vi "Post-Processing Main.vi"() -> ()   [LabVIEW 2019]
uses:
  Counts.ctl
  Post-Processing/State Data.ctl
  Post-Processing/File Entry.ctl
  Post-Processing/ADC Bounds.ctl
  <vilib>/Utility/sysdir.llb/System Directory Type.ctl
  Post-Processing/Muon Data Post-Processing.lvlib
panel:
  out "Total Duration":string
  in  "Display Type":enum16{"Both", "Nearest", "Largest"}(ring)
  out "Version Number":string
  out "Total Duration (s)":dbl
  in  "Count only matching 3-Events":bool=TRUE
  in  "File":string(combo)
  in  "Directory":path
  in  "Slave Slider":cluster{"Numeric":u16, "Numeric":u16}(slide)={"Numeric"=0, "Numeric"=1} scale=0.0..1023.0
  in  "Master Slider":cluster{"Numeric":u16, "Numeric":u16}(slide)={"Numeric"=0, "Numeric"=9} scale=0.0..1023.0
  out "Slave 'Histogram'":cluster{cluster{dbl, dbl}[]}[](graph)
  out "Master 'Histogram'":cluster{cluster{dbl, dbl}[]}[](graph)
  out "Event Counts":T1 {"Coincident Event Rate" format="%.4g"; "Single Slave Event Rate" format="%.4g"; "Single Master Event Rate" format="%.4g"}
  out "Event ADC Counts Graph":T2(graph)
  # "S-Min, Max"
  # "M-Min, Max"
  # "The histograms show both single and coincident values"
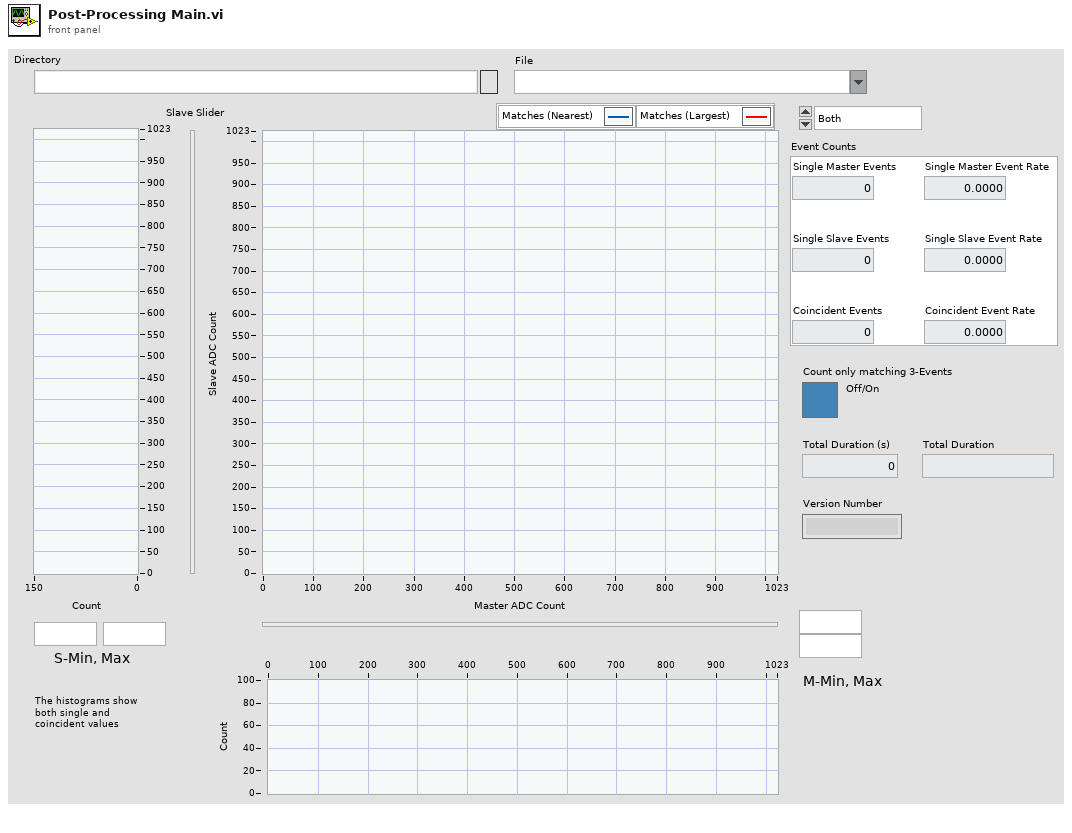
[diagram p1: front panel]
types:
  T1 = typedef "Counts.ctl" = cluster{"Single Master Events":i32, "Single Slave Events":i32, "Coincident Events":i32, "Single Master Event Rate":dbl, "Single Slave Event Rate":dbl, "Coincident Event Rate":dbl}
  T2 = cluster{"Matched ADC Values - Largest":cluster{"Master ADC Value":i32, "Slave ADC Value":i32}[]}[]
  T3 = enum32{"Invalid", "Standard", "Closed", "Hidden", "Minimized", "Maximized"}
  T4 = typedef "System Directory Type.ctl" = i32
  T5 = typedef "Muon Data Post-Processing.lvlib/State Data.ctl" = cluster{"Raw File Data":string, "Deduplicated String Array":string[][], "1-Entries":T6[], "2-Entries":T6[], "3-Entries":T6[], "Bounds":T7, "Matched ADC Values - Nearest":cluster{"Master ADC Value":i32, "Slave ADC Value":i32}[], "Match Entry Indices - Nearest":cluster{"Master Entry Index":i32, "Slave Entry Index":i32}[], "Filtered 1-Entries":T6[], "Filtered 2-Entries":T6[], "Filtered 3-Entries":T6[], "Total Duration":dbl, "Matched ADC Values - Largest":cluster{"Master ADC Value":i32, "Slave ADC Value":i32}[], "Match Entry Indices - Largest":cluster{"Master Entry Index":i32, "Slave Entry Index":i32}[]}
  T6 = typedef "Muon Data Post-Processing.lvlib/File Entry.ctl" = cluster{"Entry Index":i32, "PC Time":timestamp, "File Index":i32, "Arduino Time":i32, "ADC Value":i32, "Event Type":i32, "Detector":string}
  T7 = typedef "Muon Data Post-Processing.lvlib/ADC Bounds.ctl" = cluster{"M-Min":u16, "M-Max":u16, "S-Min":u16, "S-Max":u16}
  T8 = cluster{"Master ADC Value":i32, "Slave ADC Value":i32}[]
  T9 = cluster{"Matched ADC Values - Largest":cluster{"Master ADC Value":i32, "Slave ADC Value":i32}[]}
  T10 = cluster{"Matched ADC Values - Nearest":cluster{"Master ADC Value":i32, "Slave ADC Value":i32}[]}
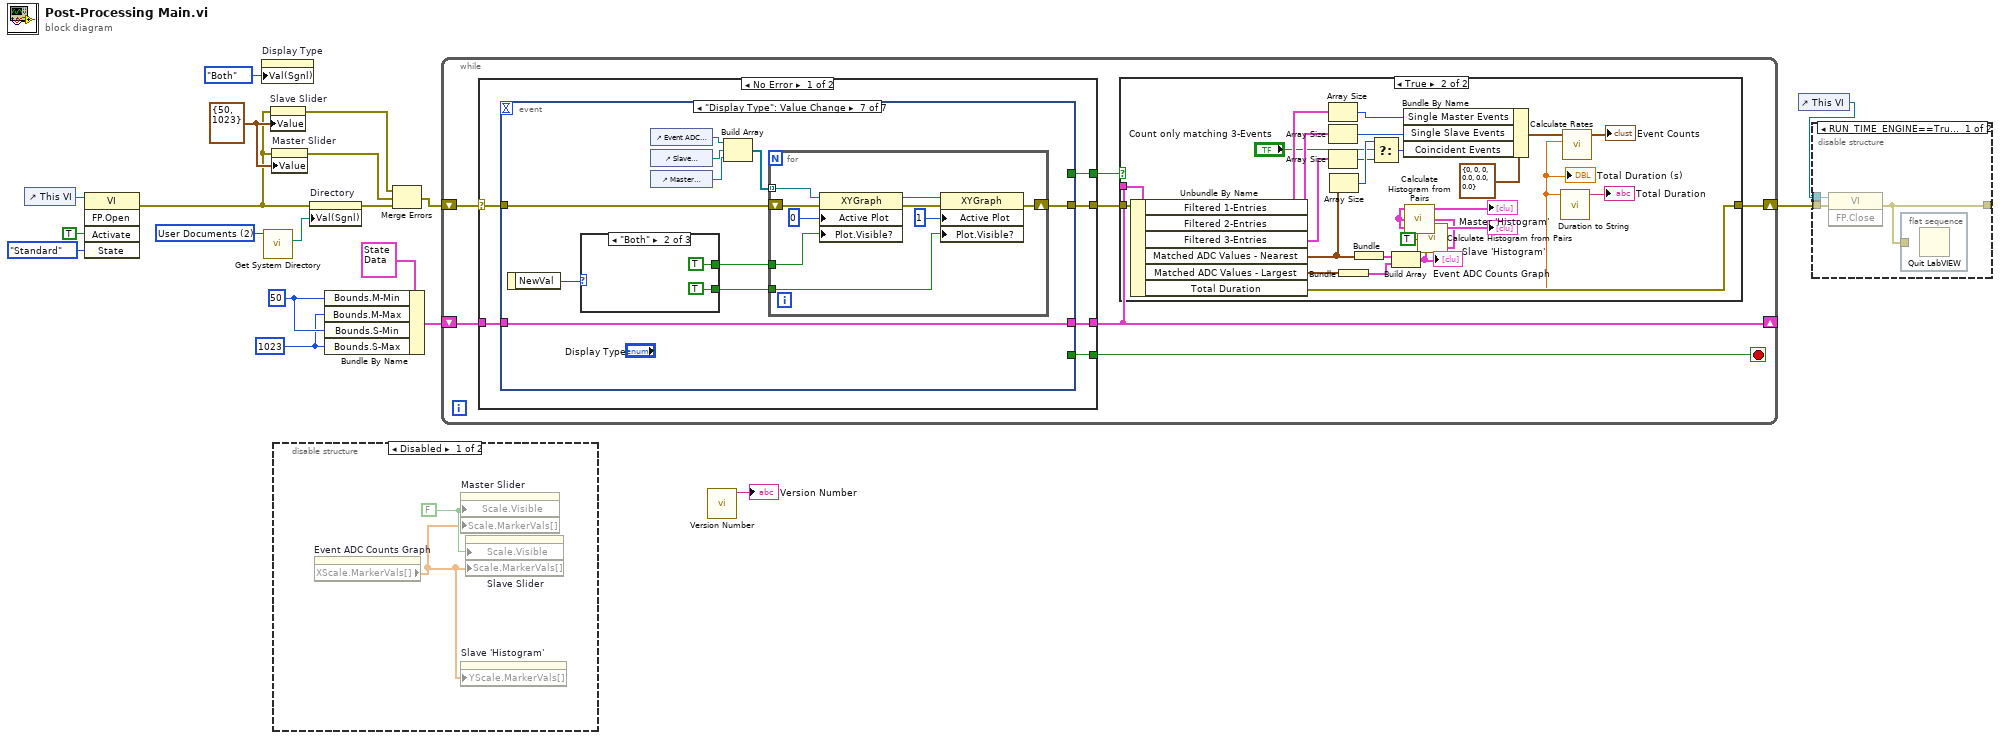
[diagram p0: block diagram]
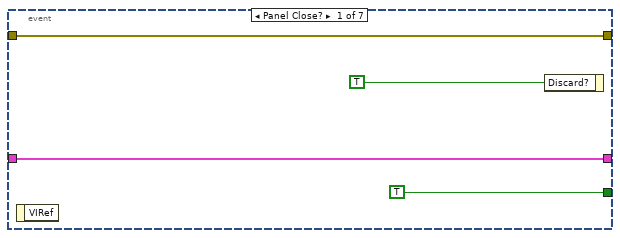
[diagram p3: hidden frame]
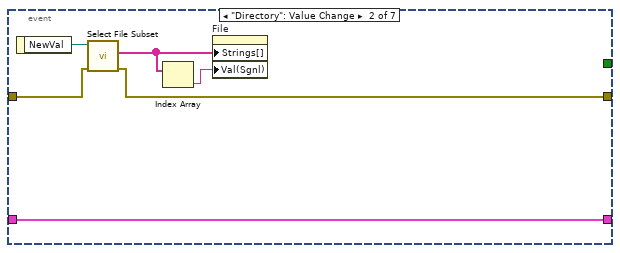
[diagram p4: hidden frame]
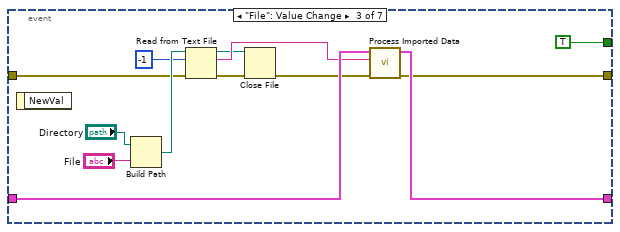
[diagram p5: hidden frame]
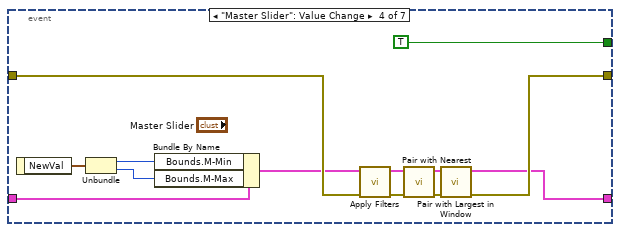
[diagram p6: hidden frame]
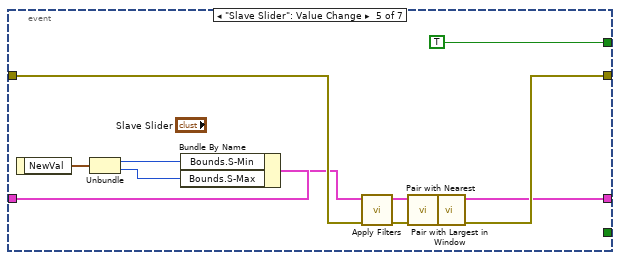
[diagram p7: hidden frame]
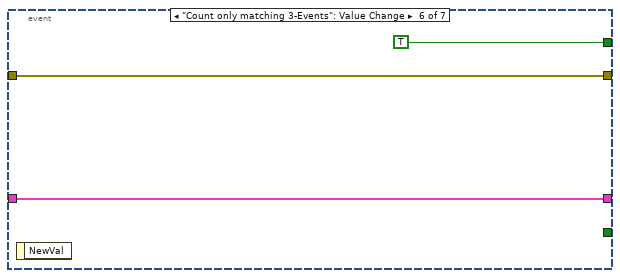
[diagram p8: hidden frame]
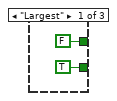
[diagram p9: hidden frame]
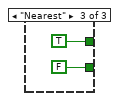
[diagram p10: hidden frame]
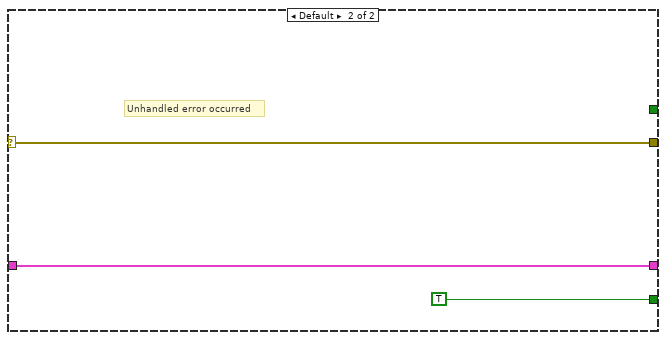
[diagram p11: hidden frame]
diagram:
  w11 = T4 2 items=["User Home"=0, "User Desktop"=1, "User Documents"=2, "User Application Data"=3, "User Preferences"=4, "User Temporary"=5, "Public Documents"=6, "Public Application Data"=7, "Public Preferences"=8, "Public Cache"=13, "System Core Libraries"=9, "System Installed Libraries"=10, "Application Files"=11, "Boot Volume Root"=12] ("system directory type")
  w12 = u16 1023 ("Bounds.M-Max")
  w13 = u16 50 ("Bounds.M-Min")
  w17 = cluster{"Numeric":u16, "Numeric":u16} {"Numeric"=50, "Numeric"=1023} ("Slave Slider")
  n1 = control-ref of="This VI"() -> (w9:refnum<vi>)
  n2 = invoke class="VI" method="FP.Open"(reference=w9, "Activate"=TRUE ("Activate?"), "State"=T3."Standard") -> (error out=w4:errorcluster)  [unwired: 2 in, 4 out]
  n3 = property on="Display Type" class="Enum (strict)"("Val(Sgnl)"=enum16{"Both", "Nearest", "Largest"}."Both" ("Value (Signaling)")) -> ()  [unwired: 2 in, 2 out]
  n4 = call <vilib>:"Get System Directory.vi"("system directory type"=w11) -> ("system directory"=w10:path)  [unwired: 10 in]
  n5 = property on="Slave Slider" class="Slide (strict)"(error in=w4, "Value"=w17) -> (error out=w16:errorcluster)  [unwired: 1 in, 1 out]
  n6 = property on="Master Slider" class="Slide (strict)"(error in=w4, "Value"=w17) -> (error out=w15:errorcluster)  [unwired: 1 in, 1 out]
  n7 = disable-structure shown="Disabled" {
    frame Disabled {
      w21 = FALSE ("Scale.Visible")
      n8 = property on="Event ADC Counts Graph" class="XYGraph (strict)"() -> ("XScale.MarkerVals[]"=w20:dbl[])  [unwired: 2 in, 2 out]
      n9 = property on="Master Slider" class="Slide (strict)"("Scale.Visible"=w21, "Scale.MarkerVals[]"=w20) -> ()  [unwired: 2 in, 2 out]
      n10 = property on="Slave 'Histogram'" class="XYGraph (strict)"("YScale.MarkerVals[]"=w20) -> ()  [unwired: 2 in, 2 out]
      n11 = property on="Slave Slider" class="Slide (strict)"("Scale.Visible"=w21, "Scale.MarkerVals[]"=w20) -> ()  [unwired: 2 in, 2 out]
    }
    frame Enabled {
    }
  }
  n12 = property on="Directory" class="Path"(error in=w4, "Val(Sgnl)"=w10) -> (error out=w19:errorcluster)  [unwired: 1 in, 1 out]
  n13 = Bundle By Name(cluster=T5 {"Raw File Data"="", "Deduplicated String Array"=[], "1-Entries"=[], "2-Entries"=[], "3-Entries"=[], "Bounds"={"M-Min"=0, "M-Max"=1023, "S-Min"=0, "S-Max"=1023}, "Matched ADC Values - Nearest"=[], "Match Entry Indices - Nearest"=[], "Filtered 1-Entries"=[], "Filtered 2-Entries"=[], "Filtered 3-Entries"=[], "Total Duration"=0.0, "Matched ADC Values - Largest"=[], "Match Entry Indices - Largest"=[]}, "Bounds.M-Min"=w13, "Bounds.M-Max"=w12, "Bounds.S-Min"=w13, "Bounds.S-Max"=w12) -> (w14:T5)
  n14 = Merge Errors(w16, w15, w19) -> (w3:errorcluster)
  n15 = while {
    shift-right: [w24] -> w6
    shift-left: w3 -> [w26]
    shift-right: [w28] -> _
    shift-left: w14 -> [w25]
    stop <- w27 stop-if-true
    n16 = case shown="No Error" w26 {
      selector: w26 -> [w33 w114]
      tunnel: [w34 TRUE] -> w27
      tunnel: [w32 w114] -> w23
      tunnel: w25 -> [w31 w112]
      tunnel: [w30 w112] -> w28
      tunnel: [w29 _] -> w22
      frame No Error {
        n17 = event shown="[6] \"Display Type\": Value Change" {
          selector: _ -> [_ _ _ _ _ _ _]
          dyn-events: _ -> [_ _ _ _ _ _ _]
          timeout: _ -> [_ _ _ _ _ _ _]
          tunnel: [TRUE _ _ _ _ _ _] -> w34
          tunnel: w33 -> [w36 w41 w52 w69 w83 w85 w94]
          tunnel: [w36 w40 w46 w60 w73 w85 w95] -> w32
          tunnel: w31 -> [w35 w39 w57 w68 w78 w84 w96]
          tunnel: [w35 w39 w48 w58 w71 w84 w96] -> w30
          tunnel: [_ _ TRUE TRUE TRUE TRUE _] -> w29
          event Panel Close? {
            n18 = event-data() -> ()  [unwired: 1 in, 1 out]
            n19 = event-data("Discard?"=TRUE) -> ()  [unwired: 1 in, 1 out]
          }
          event "Directory": Value Change {
            n20 = event-data() -> ("NewVal"=w43:path)  [unwired: 1 in]
            n21 = call "Select File Subset.vi"("error in"=w41, "Directory"=w43) -> ("error out"=w40:errorcluster, "File List"=w42:string[])  [unwired: 8 in]
            n22 = Index Array(array=w42) -> (element=w44:string)  [unwired: 1 in]
            n23 = property on="File" class="CmbBox"("Strings[]"=w42, "Val(Sgnl)"=w44) -> ()  [unwired: 2 in, 2 out]
          }
          event "File": Value Change {
            n24 = event-data() -> ()  [unwired: 1 in, 1 out]
            n25 = Build Path(base path="Directory", name or relative path="File") -> (appended path=w55:path)
            n26 = Read from Text File(file (use dialog)=w55, count=-1, error in=w52) -> (refnum out=w50:refnum<file>, text=w56:string, error out=w51:errorcluster)  [unwired: 1 in, 1 out]
            n27 = Close File(refnum=w50, error in=w51) -> (error out=w47:errorcluster)  [unwired: 1 out]
            n28 = call "Process Imported Data.vi"("error in (no error)"=w47, "Raw File Data"=w56, "State Data in"=w57) -> ("error out"=w46:errorcluster, "State Data out"=w48:T5)  [unwired: 7 in]
          }
          event "Master Slider": Value Change {
            n29 = event-data() -> ("NewVal"=w66:cluster{"Numeric":u16, "Numeric":u16})  [unwired: 1 in]
            n30 = Unbundle(w66) -> ("Numeric"=w65:u16, "Numeric"=w64:u16)
            n31 = Bundle By Name(cluster=w68, "Bounds.M-Min"=w65, "Bounds.M-Max"=w64) -> (w62:T5)
            n32 = call "Apply Filters.vi"("error in (no error)"=w69, "State in"=w62) -> ("error out"=w63:errorcluster, "State out"=w61:T5)  [unwired: 8 in]
            n33 = call "Pair with Nearest.vi"("error in (no error)"=w63, "State in"=w61) -> ("error out"=w70:errorcluster, "State out"=w59:T5)  [unwired: 8 in]
            n34 = call "Pair with Largest in Window.vi"("error in (no error)"=w70, "State in"=w59) -> ("error out"=w60:errorcluster, "State out"=w58:T5)  [unwired: 8 in]
          }
          event "Slave Slider": Value Change {
            n35 = event-data() -> ("NewVal"=w79:cluster{"Numeric":u16, "Numeric":u16})  [unwired: 1 in]
            n36 = Unbundle(w79) -> ("Numeric"=w81:u16, "Numeric"=w80:u16)
            n37 = Bundle By Name(cluster=w78, "Bounds.S-Min"=w81, "Bounds.S-Max"=w80) -> (w75:T5)
            n38 = call "Apply Filters.vi"("error in (no error)"=w83, "State in"=w75) -> ("error out"=w76:errorcluster, "State out"=w74:T5)  [unwired: 8 in]
            n39 = call "Pair with Nearest.vi"("error in (no error)"=w76, "State in"=w74) -> ("error out"=w82:errorcluster, "State out"=w72:T5)  [unwired: 8 in]
            n40 = call "Pair with Largest in Window.vi"("error in (no error)"=w82, "State in"=w72) -> ("error out"=w73:errorcluster, "State out"=w71:T5)  [unwired: 8 in]
          }
          event "Count only matching 3-Events": Value Change {
            n41 = event-data() -> ()  [unwired: 1 in, 1 out]
          }
          event "Display Type": Value Change {
            n42 = event-data() -> ("NewVal"=w93:enum16{"Both", "Nearest", "Largest"})  [unwired: 1 in]
            n43 = case shown="\"Both\"" w93 {
              tunnel: [TRUE TRUE FALSE] -> w92
              tunnel: [FALSE TRUE TRUE] -> w91
              frame "Largest" {
              }
              frame "Both" {
              }
              frame "Nearest" {
              }
            }
            n44 = control-ref of="Event ADC Counts Graph"() -> (w90:refnum<vi>)
            n45 = control-ref of="Slave 'Histogram'"() -> (w89:refnum<vi>)
            n46 = control-ref of="Master 'Histogram'"() -> (w88:refnum<vi>)
            n47 = Build Array(w90, w89, w88) -> (w87:refnum<vi>[])
            n48 = for {
              tunnel: w92 -> [w100]
              tunnel: w91 -> [w99]
              shift-right: [w102] -> w95
              shift-left: w94 -> [w101]
              tunnel: w87 -> [w97] mode=indexing
              n49 = property on="Property Node" class="XYGraph"(reference=w97, error in=w101, "Active Plot"=u32 0, "Plot.Visible?"=w99) -> (reference out=w98:refnum<vi>, error out=w103:errorcluster)
              n50 = property on="Property Node" class="XYGraph"(reference=w98, error in=w103, "Active Plot"=u32 1, "Plot.Visible?"=w100) -> (error out=w102:errorcluster)  [unwired: 1 out]
            }
          }
        }
      }
      frame Default {
        # "Unhandled error occurred"
      }
    }
    n51 = case shown="True" w22 {
      tunnel: [w115 w139] -> w24
      tunnel: w23 -> [w115 w139]
      tunnel: w28 -> [_ w138]
      frame False {
      }
      frame True {
        w118 = TRUE ("Switch X/Y")
        n52 = Unbundle By Name(w138) -> ("Filtered 1-Entries"=w137:T6[], "Filtered 2-Entries"=w135:T6[], "Filtered 3-Entries"=w136:T6[], "Matched ADC Values - Nearest"=w117:T8, "Matched ADC Values - Largest"=w125:T8, "Total Duration"=w122:dbl)
        "Total Duration (s)" <- w122
        n53 = Array Size(array=w137) -> (size(s)=w133:i32)
        n54 = Array Size(array=w135) -> (size(s)=w132:i32)
        n55 = Array Size(array=w136) -> (size(s)=w128:i32)
        n56 = Array Size(array=w117) -> (size(s)=w129:i32)
        n57 = Bundle("Matched ADC Values - Largest"=w125) -> (w123:T9)  [unwired: 1 in]
        n58 = Bundle("Matched ADC Values - Nearest"=w117) -> (w124:T10)  [unwired: 1 in]
        n59 = Select(t=w129, s="Count only matching 3-Events", f=w128) -> (s? t:f=w127:i32)
        n60 = Build Array(w124, w123) -> (w116:T2)
        "Event ADC Counts Graph" <- w116
        n61 = Bundle By Name(cluster=T1 {"Single Master Events"=0, "Single Slave Events"=0, "Coincident Events"=0, "Single Master Event Rate"=0.0, "Single Slave Event Rate"=0.0, "Coincident Event Rate"=0.0} ("Event Counts"), "Single Master Events"=w133, "Single Slave Events"=w132, "Coincident Events"=w127) -> (w131:T1)
        n62 = call "Calculate Histogram from Pairs.vi"("Matched Values"=w116) -> ("Histogram Data"=→"Master 'Histogram'":cluster{cluster{dbl, dbl}[]}[])  [unwired: 10 in]
        n63 = call "Calculate Histogram from Pairs.vi"("Slave Histogram"=w118, "Switch X/Y"=w118, "Matched Values"=w116) -> ("Histogram Data"=→"Slave 'Histogram'":cluster{cluster{dbl, dbl}[]}[])  [unwired: 8 in]
        n64 = call "Duration to String.vi"("Duration (s)"=w122) -> ("Duration String"=→"Total Duration":string)  [unwired: 10 in]
        n65 = call "Calculate Rates.vi"("Duration (s)"=w122, "Event Counts"=w131) -> ("Event Counts with Rate"=→"Event Counts":T1)  [unwired: 9 in]
      }
    }
  }
  n66 = call "Version Number.vi"() -> ("Version Number"=→"Version Number":string)  [unwired: 11 in]
  n67 = control-ref of="This VI"() -> (w5:refnum<vi>)
  n68 = disable-structure shown="RUN_TIME_ENGINE==True" {
    disable-tunnel: w6 -> [w142 w143]
    disable-tunnel: [w140 w143] -> _
    disable-tunnel: w5 -> [w141 _]
    frame condition #0 {
      n69 = invoke class="VI" method="FP.Close"(reference=w141, error in=w142) -> (error out=w140:errorcluster)  [unwired: 1 in, 2 out]
      n70 = flat-sequence {
        tunnel: w140 -> [_]
        frame #0 {
          n71 = Quit LabVIEW() -> ()  [unwired: 1 in]
        }
      }
    }
    frame condition #1 (active) {
    }
  }
